vi "Upload Part.vi"(7 "Content MD5":string, 8 "error in (no error)":errorcluster, 9 "Part Number":u16=1 min=1 max=10000, 10 "Data":string, 11 "Multipart Upload RefNum in":T1) -> (0 "error out":errorcluster, 2 "Success?":bool, 3 "Multipart Upload RefNum out":T1)   [LabVIEW 2011, in "LV Interface for Amazon S3.lvlib"]
doc: "This operation <B>uploads a part in a multipart upload</B>. <B>You must initiate a multipart upload</B> (see Initiate Multipart Upload.vi) <B>before you can upload any part</B>. In response to your initiate request, you will receive a Multipart Upload Refnum, that you must use through the whole upload process."
uses:
  LV Interface for Amazon S3.lvlib
  Typedefs/AMZ_S3_Multipart Upload RefNum.ctl
  Typedefs/AMZ_S3_Multipart Upload RefNum Enum.ctl
  Typedefs/AMZ_S3_HTTP Header-Value pair.ctl
  Typedefs/AMZ_S3_Multipart Upload Part Data.ctl
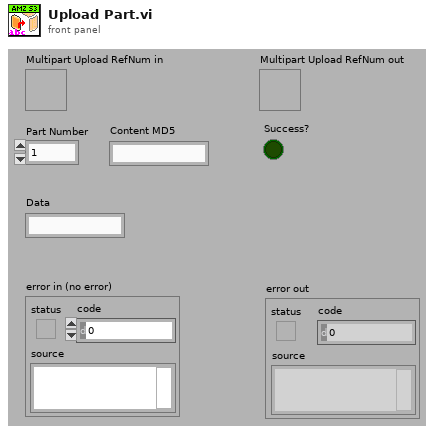
[diagram p1: front panel]
types:
  T1 = typedef "LV Interface for Amazon S3.lvlib/AMZ_S3_Multipart Upload RefNum.ctl" = refnum<k1>
  T2 = typedef "LV Interface for Amazon S3.lvlib/AMZ_S3_Multipart Upload Data.ctl" = cluster{"Object":string, "Bucket":string, "UploadID":string, "Parts":T3[]}
  T3 = typedef "LV Interface for Amazon S3.lvlib/AMZ_S3_Multipart Upload Part Data.ctl" = cluster{"PartNumber":u16, "Lat modified":timestamp, "ETag":string, "Size":u64}
  T4 = typedef "LV Interface for Amazon S3.lvlib/AMZ_S3_HTTP Header-Value pair.ctl" = cluster{"Header":string, "Value":string}
  T5 = typedef "LV Interface for Amazon S3.lvlib/AMZ_S3_Call Results.ctl" = enum16{"Success", "UndefinedError", "AccessDenied", "AccountProblem", "AmbiguousGrantByEmailAddress", "BadDigest", "BucketAlreadyExists", "BucketAlreadyOwnedByYou", "BucketNotEmpty", "CredentialsNotSupported", "CrossLocationLoggingProhibited", "EntityTooSmall", "EntityTooLarge", "ExpiredToken", "IllegalVersioningConfigurationException", "IncompleteBody", "IncorrectNumberOfFilesInPostRequest", "InlineDataTooLarge", "InternalError", "InvalidAccessKeyId", "InvalidAddressingHeader", "InvalidArgument", "InvalidBucketName", "InvalidDigest", "InvalidLocationConstraint", "InvalidPart", "InvalidPartOrder", "InvalidPayer", "InvalidPolicyDocument", "InvalidRange", "InvalidSecurity", "InvalidSOAPRequest", "InvalidStorageClass", "InvalidTargetBucketForLogging", "InvalidToken", "InvalidURI", "KeyTooLong", "MalformedACLError", "MalformedPOSTRequest", "MalformedXML", "MaxMessageLengthExceeded", "MaxPostPreDataLengthExceededError", "MetadataTooLarge", "MethodNotAllowed", "MissingAttachment", "MissingContentLength", "MissingRequestBodyError", "MissingSecurityElement", "MissingSecurityHeader", "NoLoggingStatusForKey", "NoSuchBucket", "NoSuchKey", "NoSuchUpload", "NoSuchVersion", "NotImplemented", "NotSignedUp", "OperationAborted", "PermanentRedirect", "PreconditionFailed", "Redirect", "RequestIsNotMultiPartContent", "RequestTimeout", "RequestTimeTooSkewed", "RequestTorrentOfBucketError", "SignatureDoesNotMatch", "SlowDown", "TemporaryRedirect", "TokenRefreshRequired", "TooManyBuckets", "UnexpectedContent", "UnresolvableGrantByEmailAddress", "UserKeyMustBeSpecified", "LabVIEWError"}
  T6 = typedef "LV Interface for Amazon S3.lvlib/AMZ_S3_API_UploadPartResult.ctl" = cluster{"ETag":string}
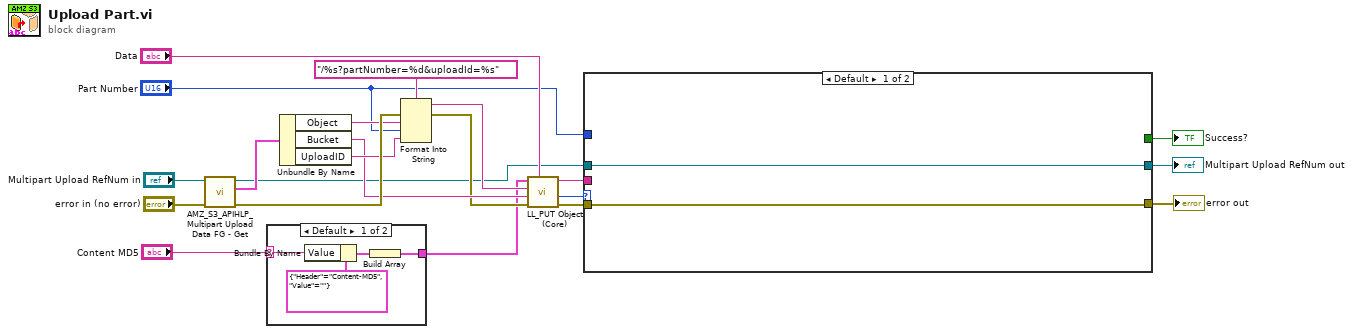
[diagram p0: block diagram]
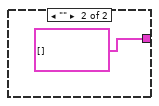
[diagram p2: hidden frame]
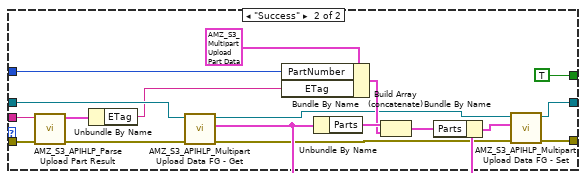
[diagram p3: hidden frame]
diagram:
  n1 = call "AMZ_S3_APIHLP_Multipart Upload Data FG - Get.vi"("error in (no error)"="error in (no error)", "Multipart Upload RefNum in"="Multipart Upload RefNum in") -> ("error out"=w18:errorcluster, "Multipart Upload Data"=w20:T2, "Multipart Upload RefNum out"=w9:T1)  [unwired: 7 in]
  n2 = case shown="Default" "Content MD5" {
    selector: "Content MD5" -> [w23 _]
    tunnel: [w22 T4[] []] -> w1
    frame Default {
      n3 = Bundle By Name(cluster=T4 {"Header"="Content-MD5", "Value"=""} ("HTTP Header-Value pair"), "Value"=w23) -> (w25:T4)
      n4 = Build Array(w25) -> (w22:T4[])
    }
    frame "" {
    }
  }
  n5 = Unbundle By Name(w20) -> ("Object"=w17:string, "Bucket"=w15:string, "UploadID"=w16:string)
  n6 = Format Into String(format string="/%s?partNumber=%d&uploadId=%s", error in=w18, w17, "Part Number", w16) -> (resulting string=w13:string, error out=w14:errorcluster)  [unwired: 1 in]
  n7 = call "LL_PUT Object (Core).vi"("Data"="Data", "error in (no error)"=w14, "Bucket"=w15, "Path and query string"=w13, "Headers"=w1) -> ("error out"=w10:errorcluster, "Call Result"=w11:T5, "Response header"=w7:string)  [unwired: 3 in, 1 out]
  n8 = case shown="Default" w11 {
    tunnel: w10 -> [w27 w46]
    tunnel: w9 -> [w28 w42]
    tunnel: [w28 w31] -> w8
    tunnel: w7 -> [_ w45]
    tunnel: "Part Number" -> [_ w39]
    tunnel: [w27 w30] -> w4
    tunnel: [_ TRUE] -> w5
    frame Default {
    }
    frame "Success" {
      n9 = call "AMZ_S3_APIHLP_Parse Upload Part Result.vi"("error in (no error)"=w46, "Response header"=w45) -> ("error out"=w43:errorcluster, "UploadPartResult"=w44:T6)  [unwired: 8 in]
      n10 = Unbundle By Name(w44) -> ("ETag"=w38:string)
      n11 = call "AMZ_S3_APIHLP_Multipart Upload Data FG - Get.vi"("error in (no error)"=w43, "Multipart Upload RefNum in"=w42) -> ("error out"=w32:errorcluster, "Multipart Upload Data"=w35:T2, "Multipart Upload RefNum out"=w36:T1)  [unwired: 7 in]
      n12 = Bundle By Name(cluster=T3 {"PartNumber"=0, "Lat modified"=timestamp(0 s since 1904-01-01), "ETag"="", "Size"=0} ("Multipart Upload Part"), "PartNumber"=w39, "ETag"=w38) -> (w37:T3)
      n13 = Unbundle By Name(w35) -> ("Parts"=w41:T3[])
      n14 = Build Array (concatenate)(w41, w37) -> (w34:T3[])
      n15 = Bundle By Name(cluster=w35, "Parts"=w34) -> (w33:T2)
      n16 = call "AMZ_S3_APIHLP_Multipart Upload Data FG - Set.vi"("error in (no error)"=w32, "Multipart Upload Data"=w33, "Multipart Upload RefNum in"=w36) -> ("error out"=w30:errorcluster, "Multipart Upload RefNum out"=w31:T1)  [unwired: 6 in, 1 out]
    }
  }
  "Multipart Upload RefNum out" <- w8
  "Success?" <- w5
  "error out" <- w4
